vi "img.Flip.vi"(6 "flip":T1, 9 "image in":u16[][](array[numeric])) -> (1 "image out":u16[][](array[numeric]))   [LabVIEW 2020]
uses:
  _controls/flip.ctl
  <userlib>/_OpenG.lib/array/array.llb/Reverse 2D Array (U16)__ogtk.vi
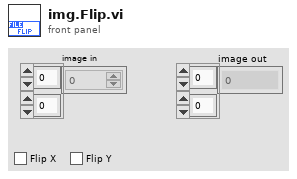
[diagram p1: front panel]
types:
  T1 = typedef "flip.ctl" = cluster{"x":bool, "y":bool}
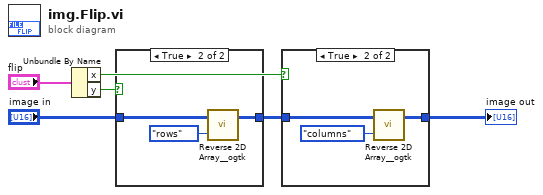
[diagram p0: block diagram]
diagram:
  n1 = Unbundle By Name("flip") -> ("x"=w3:bool, "y"=w4:bool)
  n2 = case shown="True" w4 {
    tunnel: "image in" -> [w7 w10]
    tunnel: [w7 w9] -> w2
    frame False {
    }
    frame True {
      n3 = call-poly <userlib>:"Reverse 2D Array__ogtk.vi"("by rows or columns (rows)"=enum16{"rows", "columns"}."rows", "Array"=w10) -> ("Reversed Array"=w9:u16[][])  [unwired: 1 in]
    }
  }
  n4 = case shown="True" w3 {
    tunnel: w2 -> [w11 w14]
    tunnel: [w11 w12] -> w1
    frame False {
    }
    frame True {
      n5 = call-poly <userlib>:"Reverse 2D Array__ogtk.vi"("by rows or columns (rows)"=enum16{"rows", "columns"}."columns", "Array"=w14) -> ("Reversed Array"=w12:u16[][])  [unwired: 1 in]
    }
  }
  "image out" <- w1
